vi "Send MailMessage.vi"(8 "error in (no error)":errorcluster caption="错误输入（无错误）", 11 "Email In":refnum<class "Email.lvclass"> caption="DNL_LabVIEW Object in") -> (0 "error out":errorcluster caption="错误输出", 3 "Email out":refnum<class "Email.lvclass"> caption="DNL_LabVIEW Object out")   [LabVIEW 2012, in "Email.lvclass"]
uses:
  Email.lvclass
  Email.lvclass/Email.ctl
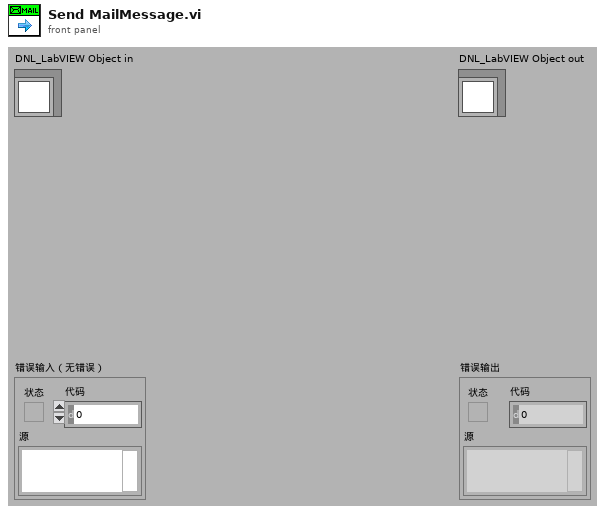
[diagram p1: front panel]
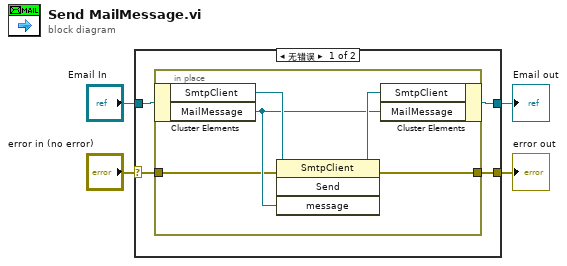
[diagram p0: block diagram]
diagram:
  n1 = case shown="无错误" "error in (no error)" {
    selector: "error in (no error)" -> [w6 w15]
    tunnel: [w5 w15] -> w3
    tunnel: [w7 w14] -> w1
    tunnel: "Email In" -> [w8 w14]
    frame No Error {
      n2 = in-place {
        in-place-border: w6 -> [w10]
        in-place-border: [w9] -> w5
        n3 = in-place-cluster #1(w8) -> ("SmtpClient"=w13:refnum<k24>, "MailMessage"=w11:refnum<k24>)
        n4 = invoke class="SmtpClient" method="Send"(reference=w13, error in=w10, "message"=w11) -> (reference out=w12:refnum<k24>, error out=w9:errorcluster)  [unwired: 1 in, 2 out]
        n5 = in-place-cluster #1("SmtpClient"=w12, "MailMessage"=w11) -> (w7:refnum<class "Email.lvclass">)
      }
    }
    frame Error {
    }
  }
  "error out" <- w3
  "Email out" <- w1
